vi "Actor Core.vi"(8 "error in":errorcluster, 11 "Threshold in":refnum<class "Threshold.lvclass">) -> (0 "error out":errorcluster, 3 "Actor out":refnum<class "Actor.lvclass">)   [LabVIEW 2016, in "Tests.lvlib" / "Threshold.lvclass"]
doc: "This VI converts RGB image into a binary image."
uses:
  Threshold.lvclass
  C:/Program Files (x86)/National Instruments/LabVIEW 2016/vi.lib/ActorFramework/Actor/Actor.lvclass
  <vilib>/ActorFramework/Actor/Actor.lvclass
  <vilib>/vision/Image Controls.llb/IMAQ Image.ctl
  Threshold Messages/New Image Threshold Msg/New Image Threshold Msg.lvclass
  C:/Users/Achu/Desktop/2015/Image Acquisition/Image Acquisition Messages/Image Msg/Image Msg.lvclass
  Controls/Threshold States.ctl
  Threshold.lvclass/Threshold.ctl
  <vilib>/ActorFramework/Actor/Actor.lvclass/Actor.ctl
  <vilib>/ActorFramework/Message Enqueuer/Message Enqueuer.lvclass/Message Enqueuer.ctl
  Controller/Controller Messages/Request Image Msg/Request Image Msg.lvclass/Request Image Msg.ctl
  <vilib>/ActorFramework/Report Error Msg/Report Error Msg.lvclass/Report Error Msg.ctl
  <vilib>/ActorFramework/Message Enqueuer/Init from Existing Queue.vi
  <vilib>/ActorFramework/Message Enqueuer/Enqueue.vi
  Controller/Controller Messages/Request Image Msg/Request Image Msg.lvclass
  C:/Program Files (x86)/National Instruments/LabVIEW 2016/vi.lib/ActorFramework/Message/Message.lvclass
  <vilib>/ActorFramework/Report Error Msg/Report Error Msg.lvclass
  Threshold Messages/Stop Threshold Actor Msg/Stop Threshold Actor Msg.lvclass
  <vilib>/ActorFramework/Stop Msg/Stop Msg.lvclass
  <vilib>/ActorFramework/Message Priority Queue/Priority Enqueue.vi
  Tests.lvclass
  <vilib>/ActorFramework/Message Enqueuer/Message Enqueuer.lvclass
  <vilib>/vision/NI_Vision_Development_Module.lvlib
panel:
  in  "Tests.lvlib:New Image Threshold Msg.lvclass":refnum<class "New Image Threshold Msg.lvclass">
  in  "Help Button":bool
  out "Thresholded Image":T1(plugin-control)
  out "New Image from Acquistion Actor":T1
  in  "Threshold Mode":enum32{"Automatic", "Manual"}(tab)
  in  "Automatic":cluster{"Object Type":u32, "Method":i32} {"Method" items=["clustering", "entropy", "metric", "moments", "inter-class variance"]; "Object Type" items=["Bright Objects", "Dark Objects"]}
  in  "Manual":cluster{sgl, sgl}(slide)={100.0, 255.0} caption="Threshold Range" scale=0.0..255.0
  out "Snapped Image":T1(plugin-control)
  in  "Apply Threshold":bool
  in  "Send Image Request":bool
  # "Threshold Viewer"
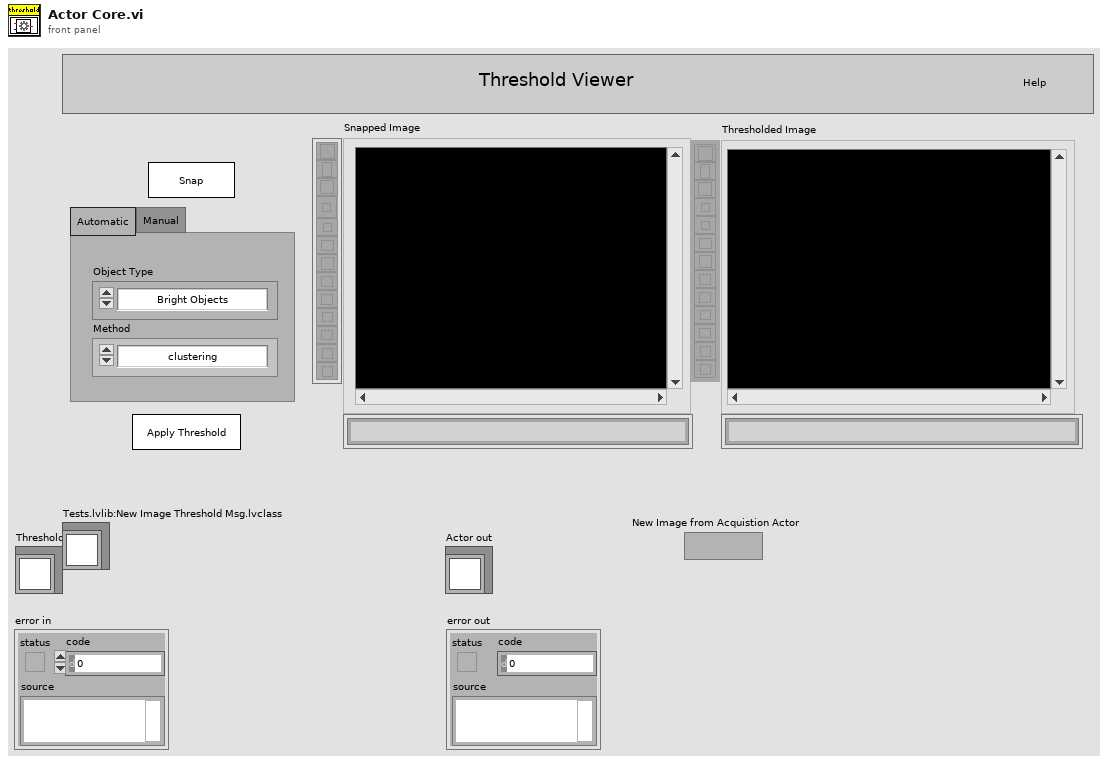
[diagram p1: front panel]
types:
  T1 = typedef "IMAQ Image.ctl" = refnum<image>
  T2 = typedef "Threshold States.ctl" = enum16{"Poll UI", "Initialize", "Send Image Request", "New Image", "Apply Threshold", "Error", "Exit"}
  T3 = enum8{"Enabled", "Disabled", "Disabled and Grayed Out"}
  T4 = typedef "Image Type" = u32
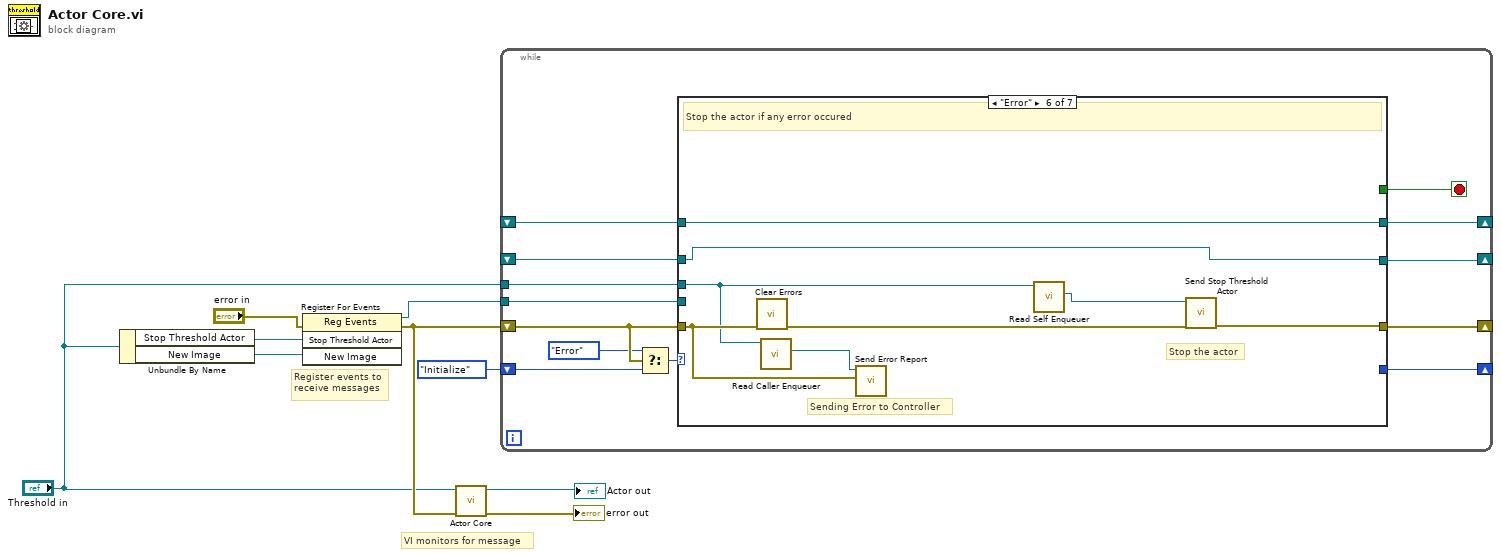
[diagram p0: block diagram]
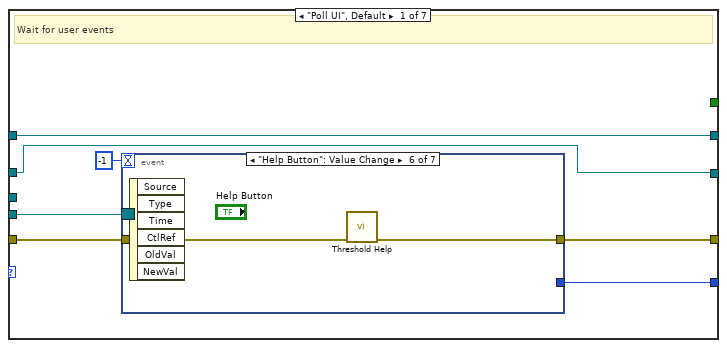
[diagram p2: hidden frame]
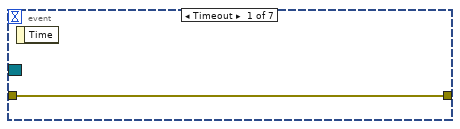
[diagram p3: hidden frame]
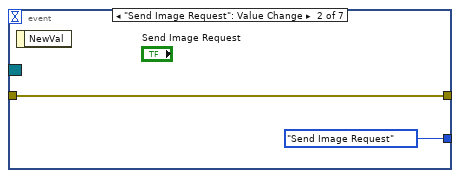
[diagram p4: hidden frame]
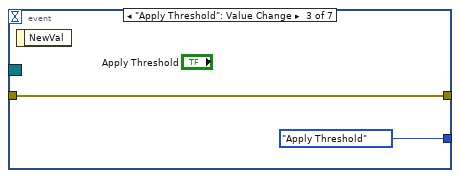
[diagram p5: hidden frame]
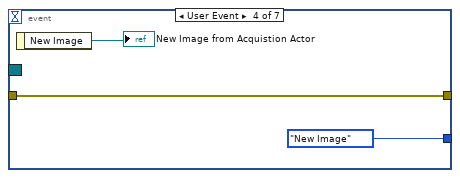
[diagram p6: hidden frame]
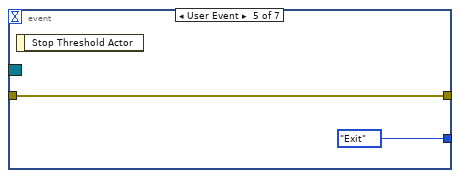
[diagram p7: hidden frame]
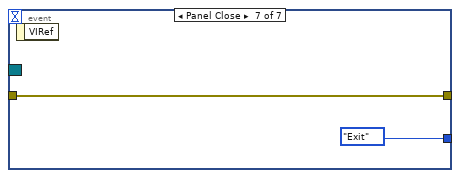
[diagram p8: hidden frame]
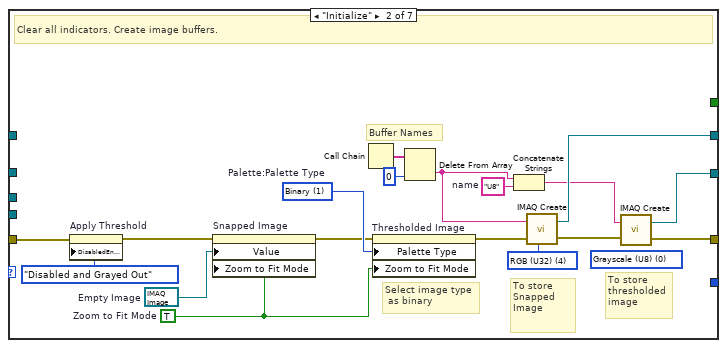
[diagram p9: hidden frame]
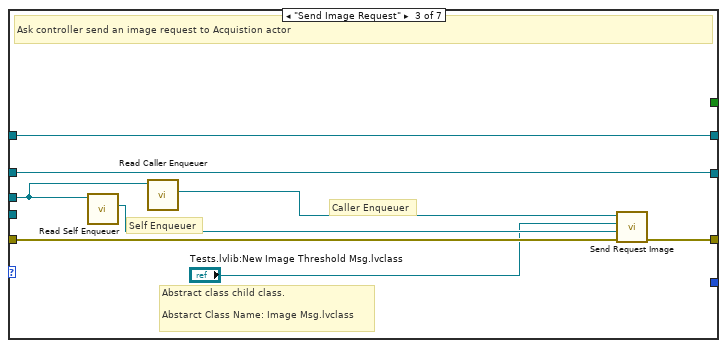
[diagram p10: hidden frame]
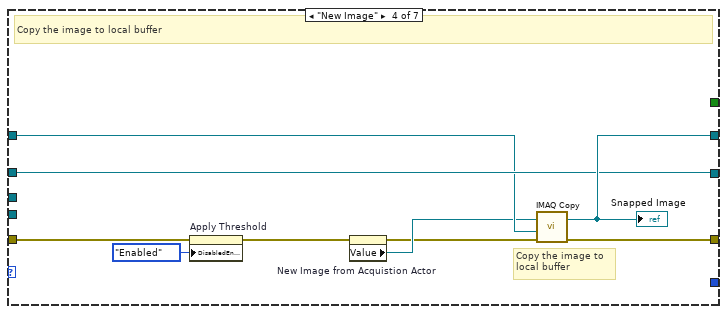
[diagram p11: hidden frame]
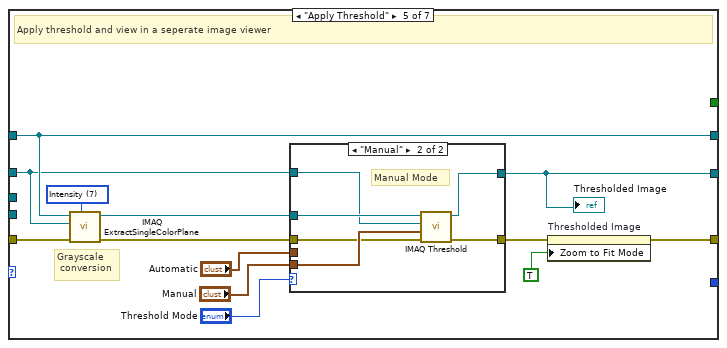
[diagram p12: hidden frame]
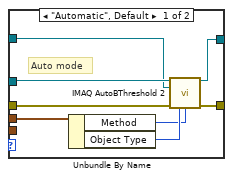
[diagram p13: hidden frame]
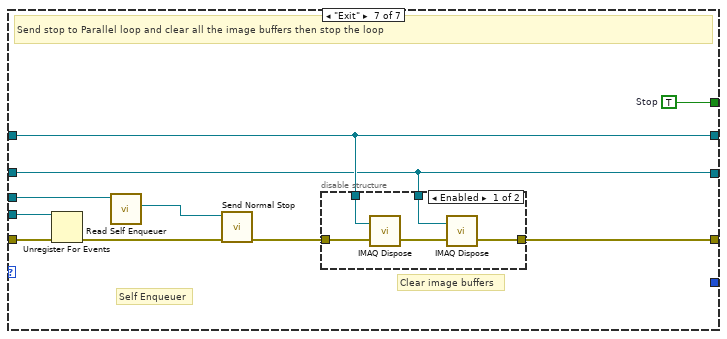
[diagram p14: hidden frame]
diagram:
  # "VI monitors for message"
  # "Register events to\nreceive messages"
  n1 = Unbundle By Name("Threshold in") -> ("Stop Threshold Actor"=w5:refnum<user-event>, "New Image"=w4:refnum<user-event>)
  n2 = register-events(error in="error in", w5, w4) -> (reference out=w7:refnum<event-registration>, error out=w2:errorcluster)  [unwired: 1 in]
  n3 = call-parent "Actor Core.vi"("error in"=w2, "Actor in"="Threshold in") -> ("error out"=→"error out":errorcluster, "Actor out"=→"Actor out":refnum<class "Actor.lvclass">)  [unwired: 8 in]
  n4 = while {
    tunnel: w7 -> [w22]
    shift-right: [w21] -> _
    shift-left: w2 -> [w19]
    shift-right: [w20] -> _
    shift-left: Threshold_States."Initialize" -> [w18]
    tunnel: "Threshold in" -> [w16]
    shift-right: [w14] -> _
    shift-left: _ -> [w13]
    shift-right: [w11] -> _
    shift-left: _ -> [w10]
    stop <- w15 stop-if-true
    n5 = Select(t=Threshold_States."Error", s=w19, f=w18) -> (s? t:f=w17:T2)
    n6 = case shown="\"Error\"" w17 {
      tunnel: w22 -> [w29 _ _ _ _ _ w120]
      tunnel: w19 -> [w28 w60 w66 w76 w91 w112 w119]
      tunnel: [w27 w54 w65 w78 w79 w107 w115] -> w21
      tunnel: [w26 _ _ _ _ _ _] -> w20
      tunnel: w16 -> [_ _ w69 _ _ w110 w123]
      tunnel: [_ _ _ _ _ _ w121] -> w15
      tunnel: [w24 w53 w64 w77 w85 w111 w117] -> w14
      tunnel: w13 -> [w24 _ w64 w73 w85 w111 w117]
      tunnel: [w25 w52 w63 w74 w82 w109 w114] -> w11
      tunnel: w10 -> [w25 _ w63 w74 w83 w109 w114]
      frame "Poll UI", Default {
        # "Wait for user events"
        n7 = event shown="[5] \"Help Button\": Value Change" {
          selector: w29 -> [_ _ _ _ _ _ _]
          dyn-events: _ -> [_ _ _ _ _ _ _]
          timeout: -1 -> [_ _ _ _ _ _ _]
          tunnel: w28 -> [w30 w32 w34 w37 w39 w41 w43]
          tunnel: [w30 w32 w34 w37 w39 w40 w43] -> w27
          tunnel: [_ Threshold_States."Send Image Request" Threshold_States."Apply Threshold" Threshold_States."New Image" Threshold_States."Exit" _ Threshold_States."Exit"] -> w26
          event Timeout {
            n8 = event-data() -> ()  [unwired: 1 in, 1 out]
          }
          event "Send Image Request": Value Change {
            n9 = event-data() -> ()  [unwired: 1 in, 1 out]
          }
          event "Apply Threshold": Value Change {
            n10 = event-data() -> ()  [unwired: 1 in, 1 out]
          }
          event User Event {
            n11 = event-data() -> ("New Image"=→"New Image from Acquistion Actor":T1)  [unwired: 1 in]
          }
          event User Event {
            n12 = event-data() -> ()  [unwired: 1 in, 1 out]
          }
          event "Help Button": Value Change {
            n13 = event-data() -> ()  [unwired: 1 in, 6 out]
            n14 = call "Threshold Help.vi"("error in (no error)"=w41) -> ("error out"=w40:errorcluster)  [unwired: 10 in]
          }
          event Panel Close {
            n15 = event-data() -> ()  [unwired: 1 in, 1 out]
          }
        }
      }
      frame "Initialize" {
        w44 = TRUE  # Zoom to Fit Mode
        w47 = u32 1 items=["Grayscale", "Binary", "Gradient", "Rainbow", "Temperature", "User Defined", "Binary 16 Bit", "Gradient 16 Bit", "Rainbow 16 Bit", "Temperature 16 Bit", "User Defined 16 Bit"]  # Palette:Palette Type
        w49 = "U8"  # name
        (unwired) T4 0 items=["Grayscale (U8)", "Grayscale (I16)", "Grayscale (SGL)", "Complex (CSG)", "RGB (U32)", "HSL (U32)", "RGB (U64)", "Grayscale (U16)"] ("Image Type")
        w57 = T4 4 items=["Grayscale (U8)", "Grayscale (I16)", "Grayscale (SGL)", "Complex (CSG)", "RGB (U32)", "HSL (U32)", "RGB (U64)", "Grayscale (U16)"] ("Image Type")
        w58 = T1 refnum  # Empty Image
        # "Buffer Names"
        # "Select image type\n as binary"
        # "To store \nthresholded\nimage"
        # "To store Snapped Image"
        # "Clear all indicators. Create image buffers."
        n16 = property on="Apply Threshold" class="Bool"(error in=w60, "DisabledEnum"=T3."Disabled and Grayed Out" ("Disabled")) -> (error out=w59:errorcluster)  [unwired: 1 in, 1 out]
        n17 = property on="Snapped Image" class="ImageControl"(error in=w59, "Value"=w58, "Zoom to Fit Mode"=w44) -> (error out=w46:errorcluster)  [unwired: 1 in, 1 out]
        n18 = Call Chain() -> (call chain=w56:string[])
        n19 = property on="Thresholded Image" class="ImageControl"(error in=w46, "Palette Type"=w47, "Zoom to Fit Mode"=w44) -> (error out=w45:errorcluster)  [unwired: 1 in, 1 out]
        n20 = Delete From Array(array=w56, index=0) -> (deleted portion=w50:string)  [unwired: 1 in, 1 out]
        n21 = Concatenate Strings(w50, w49) -> (w51:string)
        n22 = call "IMAQ Create"("Image Name"=w50, "Image Type"=w57, "error in (no error)"=w45) -> ("New Image"=w53:T1, "error out"=w55:errorcluster)  [unwired: 2 in]
        n23 = call "IMAQ Create"("Image Name"=w51, "error in (no error)"=w55) -> ("New Image"=w52:T1, "error out"=w54:errorcluster)  [unwired: 3 in]
      }
      frame "Send Image Request" {
        # "Abstract class child class.\n\nAbstarct Class Name: Image Msg.lvclass"
        # "Self Enqueuer"
        # "Caller Enqueuer"
        # "Ask controller send an image request to Acquistion actor"
        n24 = call <vilib>:"Read Self Enqueuer.vi"("Actor"=w69) -> ("Self Enqueuer"=w68:refnum<class "Message Enqueuer.lvclass">)  [unwired: 10 in]
        n25 = call <vilib>:"Read Caller Enqueuer.vi"("Actor"=w69) -> ("Caller Enqueuer"=w67:refnum<class "Message Enqueuer.lvclass">)  [unwired: 10 in]
        n26 = call "Send Request Image.vi"("error in (no error)"=w66, "Enqueuer"=w68, "Image Acquisition.lvlib:Image Msg.lvclass"="Tests.lvlib:New Image Threshold Msg.lvclass", "Message Enqueuer"=w67) -> ("error out"=w65:errorcluster)  [unwired: 6 in, 1 out]
      }
      frame "New Image" {
        # "Copy the image to\nlocal buffer"
        # "Copy the image to local buffer"
        n27 = property on="Apply Threshold" class="Bool"(error in=w76, "DisabledEnum"=T3."Enabled" ("Disabled")) -> (error out=w71:errorcluster)  [unwired: 1 in, 1 out]
        n28 = property on="New Image from Acquistion Actor" class="IMAQImage (strict)"(error in=w71) -> (error out=w70:errorcluster, "Value"=w72:T1)  [unwired: 1 in, 1 out]
        n29 = call "IMAQ Copy"("error in (no error)"=w70, "Image Dst"=w73, "Image Src"=w72) -> ("error out"=w78:errorcluster, "Image Dst Out"=w77:T1)  [unwired: 3 in]
        "Snapped Image" <- w77
      }
      frame "Apply Threshold" {
        w86 = 7 items=["Red", "Green", "Blue", "Hue", "Saturation", "Luminance", "Value", "Intensity"] ("Color Plane")
        # "Grayscale\n conversion"
        # "Apply threshold and view in a seperate image viewer"
        n30 = call "IMAQ ExtractSingleColorPlane"("Color Plane"=w86, "error in (no error)"=w91, "Image Dst"=w83, "Image Src"=w85) -> ("error out"=w87:errorcluster, "Image Dst Out"=w84:T1)  [unwired: 6 in]
        n31 = case shown="\"Manual\"" "Threshold Mode" {
          tunnel: "Automatic" -> [w99 _]
          tunnel: "Manual" -> [_ w105]
          tunnel: w87 -> [w96 w104]
          tunnel: [w95 w103] -> w80
          tunnel: w84 -> [w94 w102]
          tunnel: w83 -> [w92 w101]
          tunnel: [w93 w100] -> w82
          frame "Automatic", Default {
            # "Auto mode"
            n32 = Unbundle By Name(w99) -> ("Method"=w97:i32, "Object Type"=w98:u32)
            n33 = call "IMAQ AutoBThreshold 2"("Image Src"=w94, "Look For (Bright Objects)"=w98, "Method (clustering)"=w97, "Image Dst"=w92, "error in (no error)"=w96) -> ("Image Dst Out"=w93:T1, "error out"=w95:errorcluster)  [unwired: 8 in, 1 out]
          }
          frame "Manual" {
            # "Manual Mode"
            n34 = call "IMAQ Threshold"("error in (no error)"=w104, "Range"=w105, "Image Dst"=w101, "Image Src"=w102) -> ("error out"=w103:errorcluster, "Image Dst Out"=w100:T1)  [unwired: 6 in]
          }
        }
        "Thresholded Image" <- w82
        n35 = property on="Thresholded Image" class="ImageControl"(error in=w80, "Zoom to Fit Mode"=TRUE) -> (error out=w79:errorcluster)  [unwired: 1 in, 1 out]
      }
      frame "Error" {
        # "Stop the actor"
        # "Sending Error to Controller"
        # "Stop the actor if any error occured"
        n36 = call <vilib>:"Clear Errors.vi"("error in (no error)"=w112) -> ("error out"=w108:errorcluster)  [unwired: 5 in, 1 out]
        n37 = call <vilib>:"Read Caller Enqueuer.vi"("Actor"=w110) -> ("Caller Enqueuer"=w113:refnum<class "Message Enqueuer.lvclass">)  [unwired: 10 in]
        n38 = call <vilib>:"Send Error Report.vi"("Error From Sender"=w112, "Message Enqueuer"=w113) -> ()  [unwired: 9 in, 1 out]
        n39 = call <vilib>:"Read Self Enqueuer.vi"("Actor"=w110) -> ("Self Enqueuer"=w106:refnum<class "Message Enqueuer.lvclass">)  [unwired: 10 in]
        n40 = call "Send Stop Threshold Actor.vi"("error in (no error)"=w108, "Message Enqueuer"=w106) -> ("error out"=w107:errorcluster)  [unwired: 8 in, 1 out]
      }
      frame "Exit" {
        w121 = TRUE  # Stop
        # "Self Enqueuer"
        # "Clear image buffers"
        # "Send stop to Parallel loop and clear all the image buffers then stop the loop"
        n41 = Unregister For Events(event registration refnum=w120, error in=w119) -> (error out=w118:errorcluster)
        n42 = call <vilib>:"Read Self Enqueuer.vi"("Actor"=w123) -> ("Self Enqueuer"=w122:refnum<class "Message Enqueuer.lvclass">)  [unwired: 10 in]
        n43 = call <vilib>:"Send Normal Stop.vi"("error in (no error)"=w118, "Message Enqueuer"=w122) -> ("error out"=w116:errorcluster)  [unwired: 9 in]
        n44 = disable-structure shown="Enabled" {
          disable-tunnel: w117 -> [w128 _]
          disable-tunnel: w116 -> [w127 w129]
          disable-tunnel: [w125 w129] -> w115
          disable-tunnel: w114 -> [w124 _]
          frame Enabled {
            n45 = call "IMAQ Dispose"("Image"=w128, "error in (no error)"=w127) -> ("error out"=w126:errorcluster)  [unwired: 4 in]
            n46 = call "IMAQ Dispose"("Image"=w124, "error in (no error)"=w126) -> ("error out"=w125:errorcluster)  [unwired: 4 in]
          }
          frame Disabled {
          }
        }
      }
    }
  }
